vi "TestExec.Script Function Params to Path.vi"(10 "File":string, 11 "Folder":string) -> (0 "error out":errorcluster, 2 "Exists":bool, 3 "Path":path)   [LabVIEW 2019]
uses:
  <vilib>/KATE/Files/File Utils.lvlib
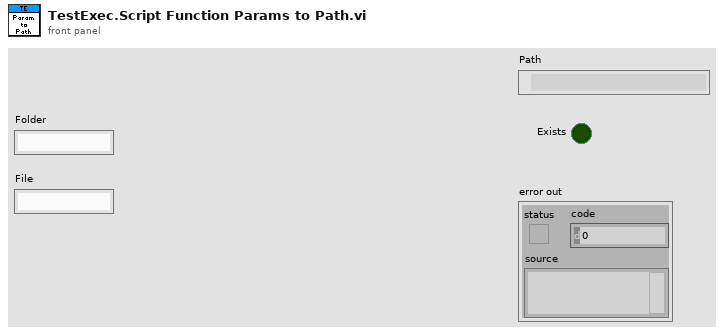
[diagram p1: front panel]
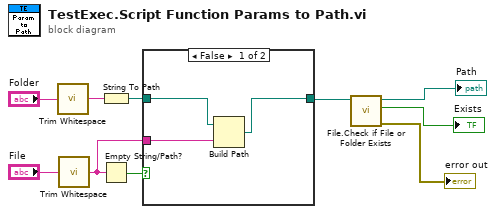
[diagram p0: block diagram]
diagram:
  n1 = call <vilib>:"Trim Whitespace.vi"("string"="Folder") -> ("trimmed string"=w7:string)  [unwired: 1 in]
  n2 = call <vilib>:"Trim Whitespace.vi"("string"="File") -> ("trimmed string"=w5:string)  [unwired: 1 in]
  n3 = String To Path(string=w7) -> (path=w6:path)
  n4 = Empty String/Path?(string/path=w5) -> (empty?=w8:bool)
  n5 = case shown="False" w8 {
    tunnel: w6 -> [w13 w14]
    tunnel: [w11 w14] -> w4
    tunnel: w5 -> [w12 _]
    frame False {
      n6 = Build Path(base path=w13, name or relative path=w12) -> (appended path=w11:path)
    }
    frame True {
    }
  }
  n7 = call <vilib>:"File.Check if File or Folder Exists.vi"("Path"=w4) -> ("error out"=→"error out":errorcluster, "Exists"=→"Exists":bool, "Dup Path"=→"Path":path)  [unwired: 6 in, 2 out]
